vi "Alternate Loop Back.vi"() -> ()   [LabVIEW 2010]
panel:
  out "Another U64 Ind":u64
  out "U8 Ind":u8
  out "U16 Ind":u16
  out "U32 Ind":u32
  out "U64 Ind":u64
  out "Another I64 Ind":i64
  out "I8 Ind":i8
  out "I16 Ind":i16
  out "I32 Ind":i32
  out "I64 Ind":i64
  in  "Another U64":u64
  in  "Another I64":i64
  in  "U8 Ctl":u8
  in  "I8 Ctl":i8
  in  "U16 Ctl":u16
  in  "I16 Ctl":i16
  in  "U32 Ctl":u32
  in  "I32 Ctl":i32
  in  "U64 Ctl":u64
  in  "I64 Ctl":i64
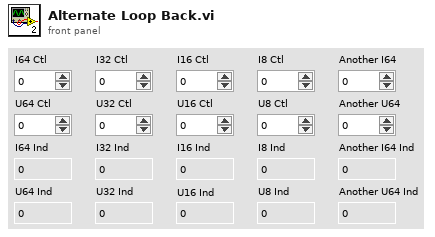
[diagram p1: front panel]
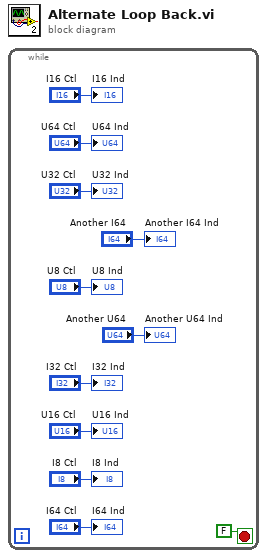
[diagram p0: block diagram]
diagram:
  n1 = while {
    stop <- FALSE stop-if-true
    "I64 Ind" <- "I64 Ctl"
    "I32 Ind" <- "I32 Ctl"
    "I16 Ind" <- "I16 Ctl"
    "I8 Ind" <- "I8 Ctl"
    "Another I64 Ind" <- "Another I64"
    "U64 Ind" <- "U64 Ctl"
    "U32 Ind" <- "U32 Ctl"
    "U16 Ind" <- "U16 Ctl"
    "U8 Ind" <- "U8 Ctl"
    "Another U64 Ind" <- "Another U64"
  }
